vi "direct_ads_dw_dp_pT.vi"(8 "Error (Input)":errorcluster, 9 "Temperature in K (Input)":dbl, 10 "Pressure in Pa (Input)":dbl, 11 "WorkingPair (Input)":T1={"no_iso"=1, "no_p_sat"=1, "path_db"="D:\\Driesel\\SorpLibLocal\\LabVIEW_wrapper\\data\\json\\sorpproplib_minimalExample.json", "wp_as"="silicagel", "wp_st"="123", "wp_iso"="DubininArctan1", "wp_rf"="water", "rf_rhol"="SaturatedLiquidDensity_EoS1", "no_rhol"=1, "rf_psat"="VaporPressure_EoS1"}) -> (0 "Error (Output)":errorcluster caption="Error(Output)", 3 "Der. of loading wrt. pressure in kg/kg/Pa (Output)":dbl)   [LabVIEW 2017]
doc: "direct_ads_dw_dp_pT:\n * --------------------\n *\n * Calculates derivative of equilibrium loading w with respect to pressure\n * p in kg/kg/Pa depending on equilibrium pressure p in Pa and equilibrium\n * temperature T in K.\n *\n * Parameters:\n * -----------\n * double p_Pa:\n * Equilibrium pressure in Pa.\n * double T_K:\n * Equilibrium temperature in K.\n *\n * const char *path_db:\n * Path to database.\n * const char *wp_as:\n * Name of sorbent.\n * const char *wp_st:\n * Name of sub-type of sorbent.\n * const char *wp_rf:\n * Name of refrigerant.\n * const char *wp_iso:\n * Name of isotherm.\n * int no_iso:\n * ID of isotherm (i.e. when more than one isotherm is available)\n * const char *rf_psat:\n * Name of calculation approach for vapor pressure.\n * int no_p_sat:\n * ID of vapor pressure equation (i.e. when more than one equation is\n * available)\n * const char *rf_rhol:\n * Name of calculation approach for liquid density.\n * int no_rhol:\n * ID of liquid density equation (i.e. when more than one equation is\n * available)\n *\n * Returns:\n * --------\n * double:\n * Derivative of equilibrium loading wrt. pressure in kg/kg/Pa.\n *\n * History:\n * --------\n * 07/06/2021, by Jannik Driesel (supervised by Mirko Engelpracht):\n * First implementation."
uses:
  data/win32bit/libsorpPropLib.dll
panel:
  # "Path to database"
  # "Name of sorbent"
  # "Name of sub-type of sorbent"
  # "Name of refrigerant"
  # "Name of isotherm"
  # "ID of isotherm"
  # "Name of calculation approach for vapor pressure"
  # "ID of vapor pressure equation"
  # "Name of calculation approach for liquid density"
  # "ID of liquid density equation"
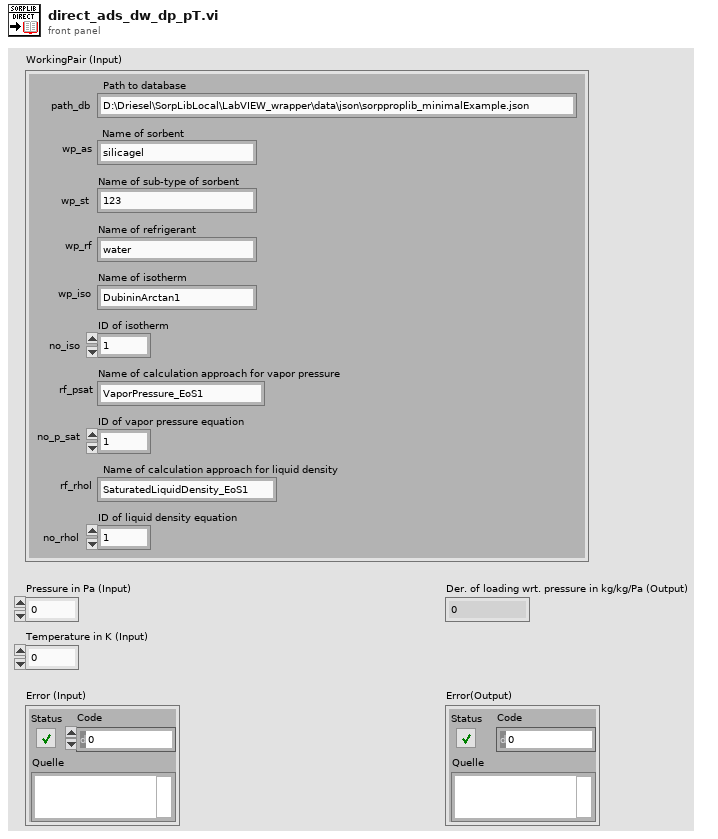
[diagram p1: front panel]
types:
  T1 = cluster{"no_iso":i32, "no_p_sat":i32, "path_db":string, "wp_as":string, "wp_st":string, "wp_iso":string, "wp_rf":string, "rf_rhol":string, "no_rhol":i32, "rf_psat":string}
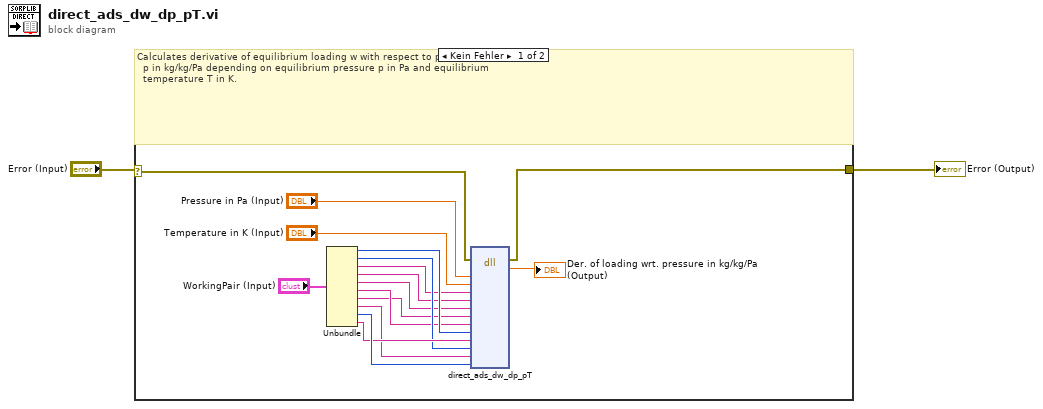
[diagram p0: block diagram]
diagram:
  n1 = case shown="Kein Fehler" "Error (Input)" {
    selector: "Error (Input)" -> [w4 w19]
    tunnel: [w3 w19] -> w1
    frame No Error {
      # "Calculates derivative of equilibrium loading w with respect to pressure\n  p in kg/kg/Pa depending on equilibrium pressure p in Pa and equilibrium\n  temperature T in K."
      n2 = Unbundle("WorkingPair (Input)") -> ("no_iso"=w12:i32, "no_p_sat"=w13:i32, "path_db"=w6:string, "wp_as"=w7:string, "wp_st"=w8:string, "wp_iso"=w10:string, "wp_rf"=w9:string, "rf_rhol"=w11:string, "no_rhol"=w15:i32, "rf_psat"=w14:string)
      n3 = dll-call lib="D:/Driesel/SorpLibLocal/LabVIEW_wrapper/data/win32bit/libsorpPropLib.dll" fn="direct_ads_dw_dp_pT"(error in=w4, "p_Pa"="Pressure in Pa (Input)", "T_K"="Temperature in K (Input)", "path_db"=w6, "wp_as"=w7, "wp_st"=w8, "wp_rf"=w9, "wp_iso"=w10, "no_iso"=w12, "rf_psat"=w14, "no_p_sat"=w13, "rf_rhol"=w11, "no_rhol"=w15) -> (error out=w3:errorcluster, "dw_dp_kgkgPa"=→"Der. of loading wrt. pressure in kg/kg/Pa (Output)":dbl)  [unwired: 14 in, 1 out]
    }
    frame Error {
      # "Error - No calculations"
    }
  }
  "Error (Output)" <- w1
